vi "module id update test.vi"() -> (0 "error out":errorcluster, 2 "Pass":bool)   [LabVIEW 2013, in "execution interface tests.lvlib"]
uses:
  execution interface tests.lvlib
  Engine Configuration/engine configuration.lvclass
  <vilib>/NI/Tag Bus/tag/Data Type.ctl
  <vilib>/NI/Tag Bus Module Framework/channel/channel classification.ctl
  <vilib>/NI/Tag Bus/tag/tag descriptor.lvclass
  <vilib>/NI/Tag Bus Module Framework/channel/TBM channel.lvclass
panel:
  out "engine configuration out":refnum<class "engine configuration.lvclass">
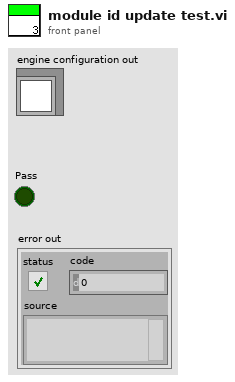
[diagram p1: front panel]
types:
  T1 = typedef "TBM channel.lvclass/channel classification.ctl" = enum16{"input data", "output data", "processing parameter", "processing result"}
  T2 = typedef "tag bus.lvlib/tag descriptor.lvclass/Data Type.ctl" = enum16{"Double", "Single", "I64", "I32", "I16", "I8", "U64", "U32", "U16", "U8", "Boolean", "String", "Array of Double", "Array of Single", "Array of I64", "Array of I32", "Array of I16", "Array of I8", "Array of U64", "Array of U32", "Array of U16", "Array of U8", "Array of Boolean", "Array of String"}
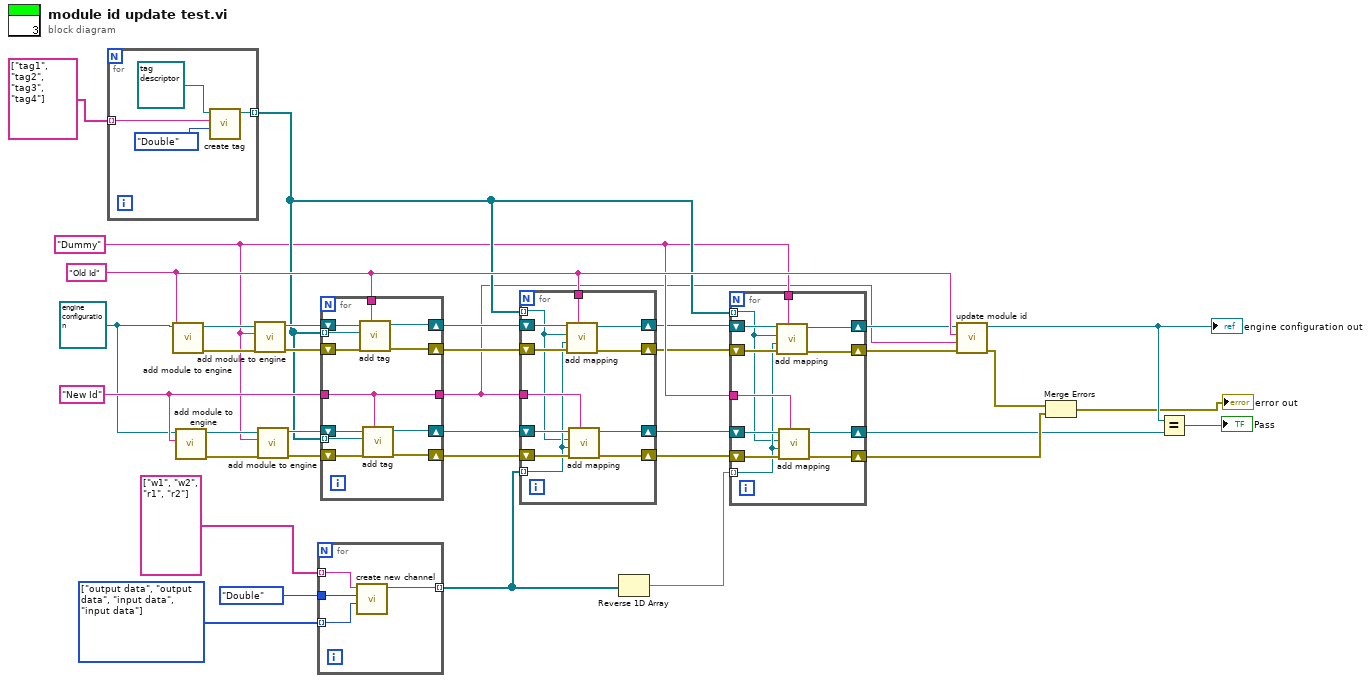
[diagram p0: block diagram]
diagram:
  w22 = T1[] [enum."output data", enum."output data", enum."input data", enum."input data"] items=["input data", "output data", "processing parameter", "processing result"]
  w28 = "New Id" ("New Id")
  w18 = "Old Id" ("Old Id")
  w12 = "Dummy" ("module ID")
  w27 = refnum<class "engine configuration.lvclass"> refnum ("engine configuration")
  n1 = for {
    tunnel: [w38] -> w13 mode=indexing
    tunnel: string[] ["tag1", "tag2", "tag3", "tag4"] -> [w37] mode=indexing
    n2 = call-dynamic "create tag.vi"("data type"=Data_Type."Double", "name"=w37, "tag descriptor in"=refnum<class "tag descriptor.lvclass"> refnum) -> ("tag descriptor out"=w38:refnum<class "tag descriptor.lvclass">)  [unwired: 7 in, 1 out]
  }
  n3 = call-dynamic "add module to engine.vi"("module ID"=w18, "engine configuration in"=w27) -> ("error out"=w34:errorcluster, "engine configuration out"=w36:refnum<class "engine configuration.lvclass">)  [unwired: 8 in]
  n4 = call-dynamic "add module to engine.vi"("module ID"=w28, "engine configuration in"=w27) -> ("error out"=w31:errorcluster, "engine configuration out"=w29:refnum<class "engine configuration.lvclass">)  [unwired: 8 in]
  n5 = call-dynamic "add module to engine.vi"("error in"=w34, "module ID"=w12, "engine configuration in"=w36) -> ("error out"=w33:errorcluster, "engine configuration out"=w35:refnum<class "engine configuration.lvclass">)  [unwired: 7 in]
  n6 = call-dynamic "add module to engine.vi"("error in"=w31, "module ID"=w12, "engine configuration in"=w29) -> ("error out"=w32:errorcluster, "engine configuration out"=w30:refnum<class "engine configuration.lvclass">)  [unwired: 7 in]
  n7 = for {
    tunnel: string[] ["w1", "w2", "r1", "r2"] -> [w42] mode=indexing
    tunnel: w22 -> [w43] mode=indexing
    tunnel: Data_Type."Double" ("data type") -> [w44]
    tunnel: [w41] -> w15 mode=indexing
    n8 = call <vilib>:"create new channel.vi"("channel classification"=w43, "data type"=w44, "channel name"=w42) -> ("channel"=w41:refnum<class "TBM channel.lvclass">)  [unwired: 8 in]
  }
  n9 = for {
    tunnel: w28 -> [w45]
    shift-right: [w49] -> w20
    shift-left: w35 -> [w56]
    shift-right: [w50] -> w17
    shift-left: w33 -> [w55]
    shift-right: [w51] -> w19
    shift-left: w30 -> [w53]
    shift-right: [w52] -> w16
    shift-left: w32 -> [w54]
    tunnel: w13 -> [w48] mode=indexing
    tunnel: w13 -> [w47] mode=indexing
    tunnel: w18 -> [w46]
    tunnel: [w45] -> w1
    n10 = call "add tag.vi"("owner ID"=w46, "error in"=w55, "tag descriptor"=w48, "engine configuration in"=w56) -> ("error out"=w50:errorcluster, "engine configuration out"=w49:refnum<class "engine configuration.lvclass">)  [unwired: 6 in]
    n11 = call "add tag.vi"("owner ID"=w45, "error in"=w54, "tag descriptor"=w47, "engine configuration in"=w53) -> ("error out"=w52:errorcluster, "engine configuration out"=w51:refnum<class "engine configuration.lvclass">)  [unwired: 6 in]
  }
  n12 = for {
    shift-right: [w65] -> w11
    shift-left: w20 -> [w68]
    shift-right: [w66] -> w9
    shift-left: w19 -> [w67]
    tunnel: w18 -> [w64]
    shift-right: [w60] -> w10
    shift-left: w17 -> [w63]
    shift-right: [w61] -> w8
    shift-left: w16 -> [w62]
    tunnel: w1 -> [w59]
    tunnel: w15 -> [w58] mode=indexing
    tunnel: w13 -> [w57] mode=indexing
    n13 = call "add mapping.vi"("owner ID"=w64, "error in"=w63, "channel"=w58, "tag descriptor"=w57, "engine configuration"=w68) -> ("error out"=w60:errorcluster, "engine configuration out"=w65:refnum<class "engine configuration.lvclass">)  [unwired: 5 in]
    n14 = call "add mapping.vi"("owner ID"=w59, "error in"=w62, "channel"=w58, "tag descriptor"=w57, "engine configuration"=w67) -> ("error out"=w61:errorcluster, "engine configuration out"=w66:refnum<class "engine configuration.lvclass">)  [unwired: 5 in]
  }
  n15 = Reverse 1D Array(array=w15) -> (reversed array=w14:refnum<class "TBM channel.lvclass">[])
  n16 = for {
    shift-right: [w77] -> w3
    shift-left: w11 -> [w80]
    shift-right: [w78] -> w2
    shift-left: w9 -> [w79]
    tunnel: w12 -> [w76]
    shift-right: [w72] -> w7
    shift-left: w10 -> [w75]
    shift-right: [w73] -> w6
    shift-left: w8 -> [w74]
    tunnel: w12 -> [w71]
    tunnel: w14 -> [w70] mode=indexing
    tunnel: w13 -> [w69] mode=indexing
    n17 = call "add mapping.vi"("owner ID"=w76, "error in"=w75, "channel"=w70, "tag descriptor"=w69, "engine configuration"=w80) -> ("error out"=w72:errorcluster, "engine configuration out"=w77:refnum<class "engine configuration.lvclass">)  [unwired: 5 in]
    n18 = call "add mapping.vi"("owner ID"=w71, "error in"=w74, "channel"=w70, "tag descriptor"=w69, "engine configuration"=w79) -> ("error out"=w73:errorcluster, "engine configuration out"=w78:refnum<class "engine configuration.lvclass">)  [unwired: 5 in]
  }
  n19 = call "update module id.vi"("error in (no error)"=w7, "New Id"=w1, "Old Id"=w18, "engine configuration in"=w3) -> ("error out"=w4:errorcluster, "engine configuration out"=w26:refnum<class "engine configuration.lvclass">)  [unwired: 6 in]
  "engine configuration out" <- w26
  n20 = Merge Errors(w4, w6) -> (→"error out":errorcluster)
  n21 = Equal?(x=w26, y=w2) -> (x = y?=→"Pass":bool)
